vi "config_test.vi"() -> ()   [LabVIEW 2015]
panel:
  in  "Tab Control":enum32{"Page 1", "Page 2"}(tab)
  in  "x":dbl
  in  "y":dbl
  out "x+y":dbl
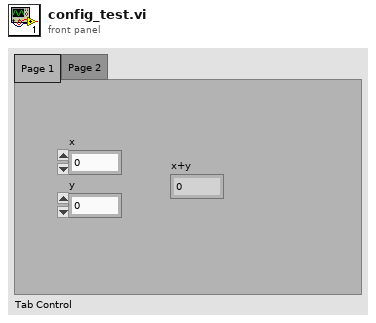
[diagram p1: front panel]
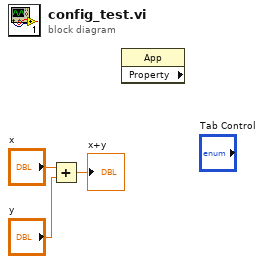
[diagram p0: block diagram]
diagram:
  n1 = Add(x="x", y="y") -> (x+y=→"x+y":dbl)
  n2 = property class="App" props=[]() -> ()  [unwired: 2 in, 3 out]
